vi "Table-Get header string.vi"(8 "error in (no error)":errorcluster, 9 "Row/Column":enum16{"Row header", "Column header"}(ring), 11 "Table":refnum<vi>) -> (0 "error out":errorcluster, 1 "Column header":string caption="Header string", 3 "Table out":refnum<vi>)   [LabVIEW 2013]
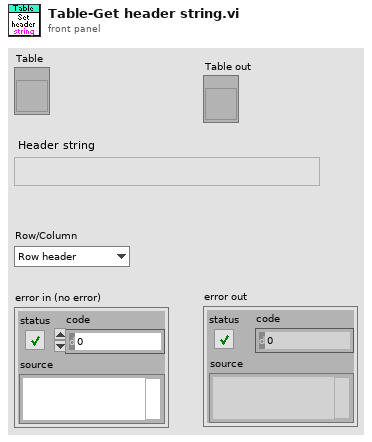
[diagram p1: front panel]
types:
  T1 = typedef "LVRowAndColumnTypeDef.ctl" = cluster{"Row":i32, "Column":i32}
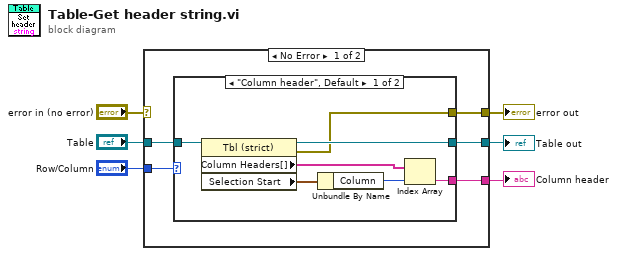
[diagram p0: block diagram]
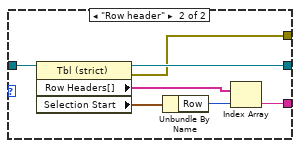
[diagram p2: hidden frame]
diagram:
  n1 = case shown="No Error" "error in (no error)" {
    selector: "error in (no error)" -> [_ w27]
    tunnel: "Table" -> [w11 w26]
    tunnel: [w10 _] -> w5
    tunnel: [w9 w26] -> w4
    tunnel: "Row/Column" -> [w8 _]
    tunnel: [w7 w27] -> w1
    frame No Error {
      n2 = case shown="\"Column header\", Default" w8 {
        tunnel: w11 -> [w18 w25]
        tunnel: [w14 w21] -> w10
        tunnel: [w13 w20] -> w9
        tunnel: [w12 w19] -> w7
        frame "Column header", Default {
          n3 = property class="Tbl (strict)"(reference=w18) -> (reference out=w13:refnum<vi>, error out=w12:errorcluster, "Column Headers[]"=w16:string[], "Selection Start"=w17:T1)  [unwired: 1 in]
          n4 = Unbundle By Name(w17) -> ("Column"=w15:i32)
          n5 = Index Array(array=w16, index=w15) -> (element=w14:string)
        }
        frame "Row header" {
          n6 = property class="Tbl (strict)"(reference=w25) -> (reference out=w20:refnum<vi>, error out=w19:errorcluster, "Row Headers[]"=w23:string[], "Selection Start"=w24:T1)  [unwired: 1 in]
          n7 = Unbundle By Name(w24) -> ("Row"=w22:i32)
          n8 = Index Array(array=w23, index=w22) -> (element=w21:string)
        }
      }
    }
    frame Error {
    }
  }
  "Column header" <- w5
  "Table out" <- w4
  "error out" <- w1
